vi "RSZVB Set UI Direction.vi"(8 "error in (no error)":errorcluster {"code" format="%.0x"}, 9 "Direction (Input)":i32(ring) items=["Input", "Output"], 10 "Port (A)":i32(ring) items=["A", "B", "C", "D"], 11 "VISA session":refnum<visa-resource-name>) -> (0 "error out":errorcluster {"code" format="%.0x"}, 3 "dup VISA session":refnum<visa-resource-name>)   [LabVIEW 2011]
doc: "This VI controls the direction of the data flow at ports A, B, C, D. The direction at the combined ports E and F is according to the configuration at the other ports.\n\nRemote-control command(s):\nCONTrol:HANDler:A:MODE INPut | OUTPut\nCONTrol:HANDler:B:MODE INPut | OUTPut\nCONTrol:HANDler:C:MODE INPut | OUTPut\nCONTrol:HANDler:D:MODE INPut | OUTPut"
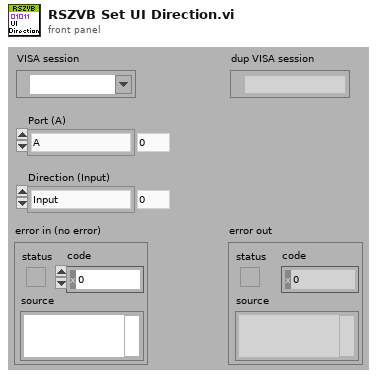
[diagram p1: front panel]
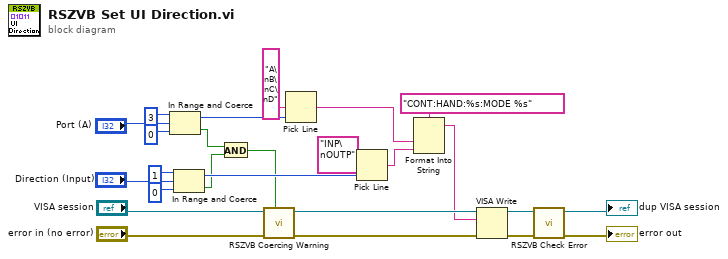
[diagram p0: block diagram]
diagram:
  n1 = In Range and Coerce(upper limit=3, x="Port (A)", lower limit=0) -> (coerced(x)=w5:i32, In Range?=w2:bool)
  n2 = In Range and Coerce(upper limit=1, x="Direction (Input)", lower limit=0) -> (coerced(x)=w16:i32, In Range?=w3:bool)
  n3 = And(x=w2, y=w3) -> (x .and. y?=w1:bool)
  n4 = call "RSZVB Coercing Warning.vi"("In Range?"=w1, "error in (no error)"="error in (no error)", "VISA session"="VISA session") -> ("error out"=w21:errorcluster, "dup VISA session"=w22:refnum<visa-resource-name>)  [unwired: 7 in]
  n5 = Pick Line(multi-line string="A\nB\nC\nD", line index=w5) -> (output string=w4:string)  [unwired: 1 in]
  n6 = Pick Line(multi-line string="INP\nOUTP", line index=w16) -> (output string=w7:string)  [unwired: 1 in]
  n7 = Format Into String(format string="CONT:HAND:%s:MODE %s", w4, w7) -> (resulting string=w18:string)  [unwired: 2 in, 1 out]
  n8 = VISA Write(VISA resource name=w22, write buffer=w18, error in (no error)=w21) -> (VISA resource name out=w19:refnum<visa-resource-name>, error out=w20:errorcluster)  [unwired: 1 out]
  n9 = call "RSZVB Check Error.vi"("error in (no error)"=w20, "VISA session"=w19) -> ("error out"=→"error out":errorcluster, "dup VISA session"=→"dup VISA session":refnum<visa-resource-name>)  [unwired: 8 in]
